vi "Create ESTTL Command.vi"(8 "error in (no error)":errorcluster, 11 "Section Ptr":T4 format="%.0x") -> (0 "error out":errorcluster, 3 "Parent Ref out":T4 format="%.0x")   [LabVIEW 2015, in "DCM System Explorer.lvlib"]
uses:
  DCM System Explorer.lvlib
  <vilib>/NI Veristand/Custom Device API/Custom Device Item Ref.ctl
  <vilib>/Powertrain Controls/Device Drivers/DCM/ESTTL/RT/Setup.ctl
  <vilib>/Powertrain Controls/Device Drivers/DCM/ESTTL/FPGA/Mode.ctl
  <vilib>/Powertrain Controls/Device Drivers/DCM/ESTTL/RT/Angle Control.ctl
  <vilib>/NI Veristand/Custom Device API/Custom Device Channel Type.ctl
  Shared/DCM Properties.vi
  <vilib>/NI VeriStand/Custom Device API/Custom Device API.lvlib
  DCM Shared.lvlib
  <vilib>/Powertrain Controls/Device Drivers/DCM/ESTTL/RT/DCM - RT - ESTTL.lvlib
  <vilib>/Powertrain Controls/Device Drivers/DCM/ESTTL/FPGA/DCM - FPGA - ESTTL.lvlib
panel:
  in  "Setup":T1[](array[typedef])=[{"Mode"=enum."Off", "Polarity"=FALSE, "Frequency [Hz]"=0.0, "Duty Cycle [%]"=0.0, "TDC Offset [CAD]"=0.0, "Window Start [DBTDC]"=0.0, "Window End [DBTDC]"=0.0, "Angles"=[{"Enable"=FALSE, "Location [DBTDC]"=0.0, "Duration [s]"=0.0}, {"Enable"=FALSE, "Location [DBTDC]"=0.0, "Duration [s]"=0.0}, {"Enable"=FALSE, "Location [DBTDC]"=0.0, "Duration [s]"=0.0}, {"Enable"=FALSE, "Location [DBTDC]"=0.0, "Duration [s]"=0.0}], "Skip Fire"=FALSE, "Skip Fire Index"=0}, {"Mode"=enum."Off", "Polarity"=FALSE, "Frequency [Hz]"=0.0, "Duty Cycle [%]"=0.0, "TDC Offset [CAD]"=0.0, "Window Start [DBTDC]"=0.0, "Window End [DBTDC]"=0.0, "Angles"=[{"Enable"=FALSE, "Location [DBTDC]"=0.0, "Duration [s]"=0.0}, {"Enable"=FALSE, "Location [DBTDC]"=0.0, "Duration [s]"=0.0}, {"Enable"=FALSE, "Location [DBTDC]"=0.0, "Duration [s]"=0.0}, {"Enable"=FALSE, "Location [DBTDC]"=0.0, "Duration [s]"=0.0}], "Skip Fire"=FALSE, "Skip Fire Index"=0}, {"Mode"=enum."Off", "Polarity"=FALSE, "Frequency [Hz]"=0.0, "Duty Cycle [%]"=0.0, "TDC Offset [CAD]"=0.0, "Window Start [DBTDC]"=0.0, "Window End [DBTDC]"=0.0, "Angles"=[{"Enable"=FALSE, "Location [DBTDC]"=0.0, "Duration [s]"=0.0}, {"Enable"=FALSE, "Location [DBTDC]"=0.0, "Duration [s]"=0.0}, {"Enable"=FALSE, "Location [DBTDC]"=0.0, "Duration [s]"=0.0}, {"Enable"=FALSE, "Location [DBTDC]"=0.0, "Duration [s]"=0.0}], "Skip Fire"=FALSE, "Skip Fire Index"=0}, {"Mode"=enum."Off", "Polarity"=FALSE, "Frequency [Hz]"=0.0, "Duty Cycle [%]"=0.0, "TDC Offset [CAD]"=0.0, "Window Start [DBTDC]"=0.0, "Window End [DBTDC]"=0.0, "Angles"=[{"Enable"=FALSE, "Location [DBTDC]"=0.0, "Duration [s]"=0.0}, {"Enable"=FALSE, "Location [DBTDC]"=0.0, "Duration [s]"=0.0}, {"Enable"=FALSE, "Location [DBTDC]"=0.0, "Duration [s]"=0.0}, {"Enable"=FALSE, "Location [DBTDC]"=0.0, "Duration [s]"=0.0}], "Skip Fire"=FALSE, "Skip Fire Index"=0}, {"Mode"=enum."Off", "Polarity"=FALSE, "Frequency [Hz]"=0.0, "Duty Cycle [%]"=0.0, "TDC Offset [CAD]"=0.0, "Window Start [DBTDC]"=0.0, "Window End [DBTDC]"=0.0, "Angles"=[{"Enable"=FALSE, "Location [DBTDC]"=0.0, "Duration [s]"=0.0}, {"Enable"=FALSE, "Location [DBTDC]"=0.0, "Duration [s]"=0.0}, {"Enable"=FALSE, "Location [DBTDC]"=0.0, "Duration [s]"=0.0}, {"Enable"=FALSE, "Location [DBTDC]"=0.0, "Duration [s]"=0.0}], "Skip Fire"=FALSE, "Skip Fire Index"=0}, {"Mode"=enum."Off", "Polarity"=FALSE, "Frequency [Hz]"=0.0, "Duty Cycle [%]"=0.0, "TDC Offset [CAD]"=0.0, "Window Start [DBTDC]"=0.0, "Window End [DBTDC]"=0.0, "Angles"=[{"Enable"=FALSE, "Location [DBTDC]"=0.0, "Duration [s]"=0.0}, {"Enable"=FALSE, "Location [DBTDC]"=0.0, "Duration [s]"=0.0}, {"Enable"=FALSE, "Location [DBTDC]"=0.0, "Duration [s]"=0.0}, {"Enable"=FALSE, "Location [DBTDC]"=0.0, "Duration [s]"=0.0}], "Skip Fire"=FALSE, "Skip Fire Index"=0}, {"Mode"=enum."Off", "Polarity"=FALSE, "Frequency [Hz]"=0.0, "Duty Cycle [%]"=0.0, "TDC Offset [CAD]"=0.0, "Window Start [DBTDC]"=0.0, "Window End [DBTDC]"=0.0, "Angles"=[{"Enable"=FALSE, "Location [DBTDC]"=0.0, "Duration [s]"=0.0}, {"Enable"=FALSE, "Location [DBTDC]"=0.0, "Duration [s]"=0.0}, {"Enable"=FALSE, "Location [DBTDC]"=0.0, "Duration [s]"=0.0}, {"Enable"=FALSE, "Location [DBTDC]"=0.0, "Duration [s]"=0.0}], "Skip Fire"=FALSE, "Skip Fire Index"=0}, {"Mode"=enum."Off", "Polarity"=FALSE, "Frequency [Hz]"=0.0, "Duty Cycle [%]"=0.0, "TDC Offset [CAD]"=0.0, "Window Start [DBTDC]"=0.0, "Window End [DBTDC]"=0.0, "Angles"=[{"Enable"=FALSE, "Location [DBTDC]"=0.0, "Duration [s]"=0.0}, {"Enable"=FALSE, "Location [DBTDC]"=0.0, "Duration [s]"=0.0}, {"Enable"=FALSE, "Location [DBTDC]"=0.0, "Duration [s]"=0.0}, {"Enable"=FALSE, "Location [DBTDC]"=0.0, "Duration [s]"=0.0}], "Skip Fire"=FALSE, "Skip Fire Index"=0}, {"Mode"=enum."Off", "Polarity"=FALSE, "Frequency [Hz]"=0.0, "Duty Cycle [%]"=0.0, "TDC Offset [CAD]"=0.0, "Window Start [DBTDC]"=0.0, "Window End [DBTDC]"=0.0, "Angles"=[{"Enable"=FALSE, "Location [DBTDC]"=0.0, "Duration [s]"=0.0}, {"Enable"=FALSE, "Location [DBTDC]"=0.0, "Duration [s]"=0.0}, {"Enable"=FALSE, "Location [DBTDC]"=0.0, "Duration [s]"=0.0}, {"Enable"=FALSE, "Location [DBTDC]"=0.0, "Duration [s]"=0.0}], "Skip Fire"=FALSE, "Skip Fire Index"=0}, {"Mode"=enum."Off", "Polarity"=FALSE, "Frequency [Hz]"=0.0, "Duty Cycle [%]"=0.0, "TDC Offset [CAD]"=0.0, "Window Start [DBTDC]"=0.0, "Window End [DBTDC]"=0.0, "Angles"=[{"Enable"=FALSE, "Location [DBTDC]"=0.0, "Duration [s]"=0.0}, {"Enable"=FALSE, "Location [DBTDC]"=0.0, "Duration [s]"=0.0}, {"Enable"=FALSE, "Location [DBTDC]"=0.0, "Duration [s]"=0.0}, {"Enable"=FALSE, "Location [DBTDC]"=0.0, "Duration [s]"=0.0}], "Skip Fire"=FALSE, "Skip Fire Index"=0}, {"Mode"=enum."Off", "Polarity"=FALSE, "Frequency [Hz]"=0.0, "Duty Cycle [%]"=0.0, "TDC Offset [CAD]"=0.0, "Window Start [DBTDC]"=0.0, "Window End [DBTDC]"=0.0, "Angles"=[{"Enable"=FALSE, "Location [DBTDC]"=0.0, "Duration [s]"=0.0}, {"Enable"=FALSE, "Location [DBTDC]"=0.0, "Duration [s]"=0.0}, {"Enable"=FALSE, "Location [DBTDC]"=0.0, "Duration [s]"=0.0}, {"Enable"=FALSE, "Location [DBTDC]"=0.0, "Duration [s]"=0.0}], "Skip Fire"=FALSE, "Skip Fire Index"=0}, {"Mode"=enum."Off", "Polarity"=FALSE, "Frequency [Hz]"=0.0, "Duty Cycle [%]"=0.0, "TDC Offset [CAD]"=0.0, "Window Start [DBTDC]"=0.0, "Window End [DBTDC]"=0.0, "Angles"=[{"Enable"=FALSE, "Location [DBTDC]"=0.0, "Duration [s]"=0.0}, {"Enable"=FALSE, "Location [DBTDC]"=0.0, "Duration [s]"=0.0}, {"Enable"=FALSE, "Location [DBTDC]"=0.0, "Duration [s]"=0.0}, {"Enable"=FALSE, "Location [DBTDC]"=0.0, "Duration [s]"=0.0}], "Skip Fire"=FALSE, "Skip Fire Index"=0}, {"Mode"=enum."Off", "Polarity"=FALSE, "Frequency [Hz]"=0.0, "Duty Cycle [%]"=0.0, "TDC Offset [CAD]"=0.0, "Window Start [DBTDC]"=0.0, "Window End [DBTDC]"=0.0, "Angles"=[{"Enable"=FALSE, "Location [DBTDC]"=0.0, "Duration [s]"=0.0}, {"Enable"=FALSE, "Location [DBTDC]"=0.0, "Duration [s]"=0.0}, {"Enable"=FALSE, "Location [DBTDC]"=0.0, "Duration [s]"=0.0}, {"Enable"=FALSE, "Location [DBTDC]"=0.0, "Duration [s]"=0.0}], "Skip Fire"=FALSE, "Skip Fire Index"=0}, {"Mode"=enum."Off", "Polarity"=FALSE, "Frequency [Hz]"=0.0, "Duty Cycle [%]"=0.0, "TDC Offset [CAD]"=0.0, "Window Start [DBTDC]"=0.0, "Window End [DBTDC]"=0.0, "Angles"=[{"Enable"=FALSE, "Location [DBTDC]"=0.0, "Duration [s]"=0.0}, {"Enable"=FALSE, "Location [DBTDC]"=0.0, "Duration [s]"=0.0}, {"Enable"=FALSE, "Location [DBTDC]"=0.0, "Duration [s]"=0.0}, {"Enable"=FALSE, "Location [DBTDC]"=0.0, "Duration [s]"=0.0}], "Skip Fire"=FALSE, "Skip Fire Index"=0}, {"Mode"=enum."Off", "Polarity"=FALSE, "Frequency [Hz]"=0.0, "Duty Cycle [%]"=0.0, "TDC Offset [CAD]"=0.0, "Window Start [DBTDC]"=0.0, "Window End [DBTDC]"=0.0, "Angles"=[{"Enable"=FALSE, "Location [DBTDC]"=0.0, "Duration [s]"=0.0}, {"Enable"=FALSE, "Location [DBTDC]"=0.0, "Duration [s]"=0.0}, {"Enable"=FALSE, "Location [DBTDC]"=0.0, "Duration [s]"=0.0}, {"Enable"=FALSE, "Location [DBTDC]"=0.0, "Duration [s]"=0.0}], "Skip Fire"=FALSE, "Skip Fire Index"=0}, {"Mode"=enum."Off", "Polarity"=FALSE, "Frequency [Hz]"=0.0, "Duty Cycle [%]"=0.0, "TDC Offset [CAD]"=0.0, "Window Start [DBTDC]"=0.0, "Window End [DBTDC]"=0.0, "Angles"=[{"Enable"=FALSE, "Location [DBTDC]"=0.0, "Duration [s]"=0.0}, {"Enable"=FALSE, "Location [DBTDC]"=0.0, "Duration [s]"=0.0}, {"Enable"=FALSE, "Location [DBTDC]"=0.0, "Duration [s]"=0.0}, {"Enable"=FALSE, "Location [DBTDC]"=0.0, "Duration [s]"=0.0}], "Skip Fire"=FALSE, "Skip Fire Index"=0}] {"Skip Fire Index" max=7; "Angles"."Duration [s]" format="%#_3p"; "Frequency [Hz]" format="%#_3p"}
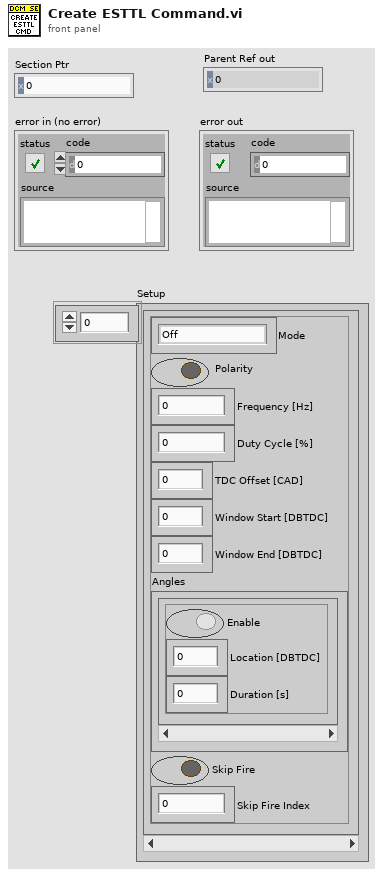
[diagram p1: front panel]
types:
  T1 = typedef "DCM - RT - ESTTL.lvlib/Setup.ctl" = cluster{"Mode":T2, "Polarity":bool, "Frequency [Hz]":sgl, "Duty Cycle [%]":sgl, "TDC Offset [CAD]":sgl, "Window Start [DBTDC]":sgl, "Window End [DBTDC]":sgl, "Angles":T3[], "Skip Fire":bool, "Skip Fire Index":u8}
  T2 = typedef "DCM - FPGA - ESTTL.lvlib/Mode.ctl" = enum8{"Off", "Pulse Width Modulation", "Engine Position Tracking"}
  T3 = typedef "DCM - RT - ESTTL.lvlib/Angle Control.ctl" = cluster{"Enable":bool, "Location [DBTDC]":sgl, "Duration [s]":sgl}
  T4 = typedef "Custom Device API.lvlib/Custom Device Item Ref.ctl" = u64
  T5 = typedef "Custom Device API.lvlib/Custom Device Channel Type.ctl" = enum16{"Input", "Output"}
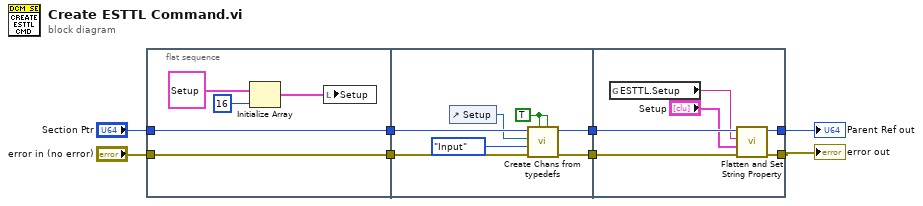
[diagram p0: block diagram]
diagram:
  n1 = flat-sequence {
    tunnel: [w12] -> w7
    tunnel: [w13] -> w8
    tunnel: "error in (no error)" -> [w13]
    tunnel: "Section Ptr" -> [w12]
    tunnel: [w16] -> w6
    tunnel: [w17] -> w5
    tunnel: w8 -> [w18]
    tunnel: w7 -> [w19]
    tunnel: [w24] -> w2
    tunnel: w6 -> [w25]
    tunnel: w5 -> [w26]
    tunnel: [w21] -> w1
    frame #0 {
      n2 = Initialize Array(T1 {"Mode"=enum."Off", "Polarity"=FALSE, "Frequency [Hz]"=0.0, "Duty Cycle [%]"=0.0, "TDC Offset [CAD]"=0.0, "Window Start [DBTDC]"=0.0, "Window End [DBTDC]"=0.0, "Angles"=[{"Enable"=FALSE, "Location [DBTDC]"=0.0, "Duration [s]"=0.0}, {"Enable"=FALSE, "Location [DBTDC]"=0.0, "Duration [s]"=0.0}, {"Enable"=FALSE, "Location [DBTDC]"=0.0, "Duration [s]"=0.0}, {"Enable"=FALSE, "Location [DBTDC]"=0.0, "Duration [s]"=0.0}], "Skip Fire"=FALSE, "Skip Fire Index"=0} ("DiffIO.Setup"), 16 ("dimension size")) -> (w11:T1[])
      n3 = local write "Setup"(w11) -> ()
    }
    frame #1 {
      w15 = TRUE ("Prevent overwrite? (F)")
      n4 = control-ref of="Setup"() -> (w14:refnum<vi>)
      n5 = call "Create Chans from typedefs.vi"("Default from text? (F)"=w15, "Prevent overwrite? (F)"=w15, "error in"=w18, "Type"=Custom_Device_Channel_Type."Input", "Ctl Ref"=w14, "Section Ref in"=w19) -> ("error out"=w17:errorcluster, "Section Ref out"=w16:T4)  [unwired: 3 in, 1 out]
    }
    frame #2 {
      n6 = global read "DCM Properties.vi" "ESTTL.Setup"() -> (w23:string)
      n7 = call "Flatten and Set String Property.vi"("error in (no error)"=w26, "Value"="Setup", "Property Name"=w23, "Section Ref in"=w25) -> ("error out"=w24:errorcluster, "Section Ref out"=w21:T4)  [unwired: 6 in]
    }
  }
  "Parent Ref out" <- w1
  "error out" <- w2
